vi "DG_Info.vi"(8 "error in (no error)":errorcluster) -> (0 "error out":errorcluster, 1 "Error code":i32, 2 "Number of Generators":i32, 3 "Generator Info":T1(array[cluster]) {"DG Product" items=["SRS_DG135"=1, "BME_DP01"=2, "BME_G02V3"=3, "BME_SG02V4"=4, "BME_G04"=5, "BME_G02V1"=6, "BME_G02V2"=7, "BME_SG02V1"=8, "BME_SG02V2"=9, "BME_SG02V3"=10, "BME_G03V1"=11, "BME_G03V2"=12, "BME_SG02V5"=13, "BME_G03V3"=14, "BME_G03V4"=15, "BME_SG02V6"=16, "BME_G03V5"=17, "BME_G05V1"=18, "BME_G05V2"=19, "BME_G05V3"=20, "BME_SG02V7"=21, "BME_SG02P1"=31, "BME_G03P1"=32, "BME_G05P1"=33, "BME_SG02P2"=34, "BME_G03P2"=35, "BME_SG02P3"=36, "BME_SG05P1"=37, "BME_G05P2"=38, "BME_SG05P2"=39, "BME_G05P3"=40, "BME_SG02P4"=41, "Unknown1"=42, "Unknown2"=43, "BME_SG08P1"=44]})   [LabVIEW 2009, in "POLARIS BME DG.lvlib"]
uses:
  POLARIS BME DG.lvlib
panel:
  # "NOTICE -- YOU MUST LEAVE THIS NOTICE IN PLACE.  PER THE TERMS OF THE LICENSE BELOW, YOU MAY SUBLICENSE THIS SOFTWARE \nIN ANY WAY THAT DOES NOT CONFLICT WITH THIS LICENSE.\n\n### BSD License (http://www.opensource.org/licenses/bsd-license.php) Begin ###\n \nCopyright (c) 2011, Applied Energetics, http://www.appliedenergetics.com,\n                               Richard Schwerdtfeger, <rschwerdtfeger@appliedenergetics.com>\n\nAll rights reserved.\n\nRedistribution and use in source and binary forms, with or without modification, are permitted provided that the \nfollowing conditions are met:\n\n    * Redistributions of source code must retain the above copyright notice, this list of conditions and the following disclaimer.\n    * Redistributions in binary form must reproduce the above copyright notice, this list of conditions and the following disclaimer \n       in the documentation and/or other materials provided with the distribution.\n    * Neither the name of Richard Schwerdtfeger, Applied Energetics, Inc., nor the names of its contributors may be used to \n       endorse or promote products derived from this software without specific prior written permission.\n\nTHIS SOFTWARE IS PROVIDED BY THE COPYRIGHT HOLDERS AND CONTRIBUTORS \"AS IS\" AND ANY EXPRESS OR IMPLIED WARRANTIES, \nINCLUDING, BUT NOT LIMITED TO, THE IMPLIED WARRANTIES OF MERCHANTABILITY AND FITNESS FOR A PARTICULAR PURPOSE ARE \nDISCLAIMED. IN NO EVENT SHALL THE COPYRIGHT OWNER OR CONTRIBUTORS BE LIABLE FOR ANY DIRECT, INDIRECT, INCIDENTAL,\n SPECIAL, EXEMPLARY, OR CONSEQUENTIAL DAMAGES (INCLUDING, BUT NOT LIMITED TO, PROCUREMENT OF SUBSTITUTE GOODS OR \nSERVICES; LOSS OF USE, DATA, OR PROFITS; OR BUSINESS INTERRUPTION) HOWEVER CAUSED AND ON ANY THEORY OF LIABILITY, \nWHETHER IN CONTRACT, STRICT LIABILITY, OR TORT (INCLUDING NEGLIGENCE OR OTHERWISE) ARISING IN ANY WAY OUT OF THE USE \nOF THIS SOFTWARE, EVEN IF ADVISED OF THE POSSIBILITY OF SUCH DAMAGE.\n\n### BSD License End ###"
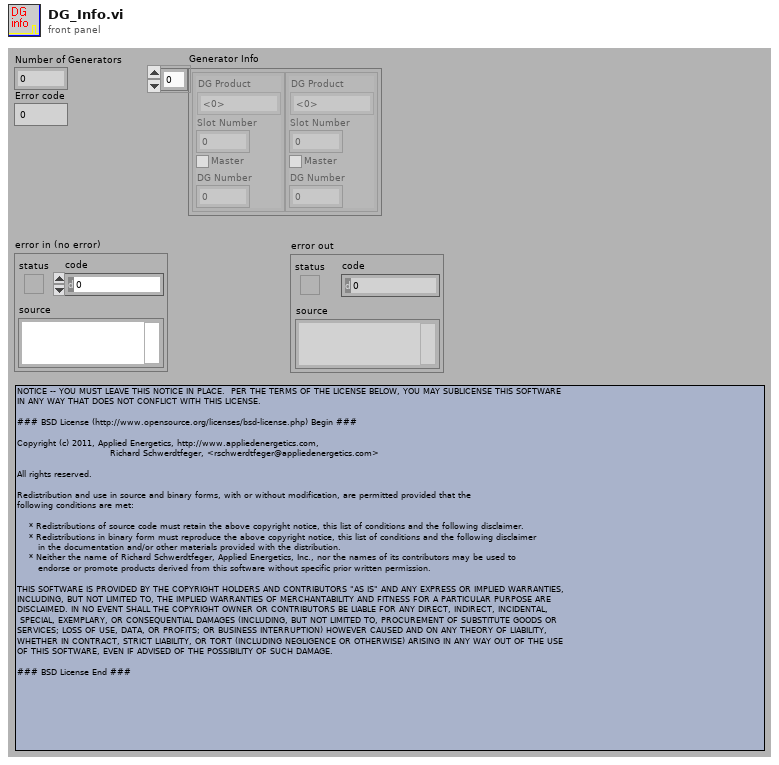
[diagram p1: front panel]
types:
  T1 = cluster{"DG Product":i32, "Slot Number":i32, "Master":bool, "DG Number":i32}[]
  T2 = cluster{"DG Product":i32, "Slot Number":i32, "Master":bool, i32}
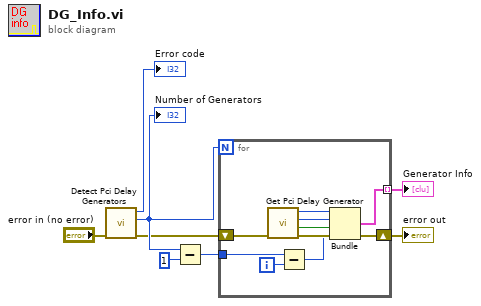
[diagram p0: block diagram]
diagram:
  n1 = call "Detect Pci Delay Generators.vi"("error in (no error)"="error in (no error)") -> ("error out"=w1:errorcluster, "Number of Generators"=w3:i32, "Error"=→"Error code":i32)  [unwired: 8 out]
  "Number of Generators" <- w3
  n2 = Subtract(x=w3, y=1) -> (x-y=w6:i32)
  n3 = for {
    N: w3 -> [_]
    tunnel: w6 -> [w16]
    tunnel: [w15] -> w8 mode=indexing
    shift-right: [w11] -> w5
    shift-left: w1 -> [w14]
    i -> [w17]
    n4 = call "Get Pci Delay Generator.vi"("error in (no error)"=w14) -> ("error out"=w11:errorcluster, "Master"=w10:bool, "Slot Number"=w12:i32, "DG Product"=w13:i32)  [unwired: 7 out]
    n5 = Subtract(x=w16, y=w17) -> (x-y=w9:i32)
    n6 = Bundle("DG Product"=w13, "Slot Number"=w12, "Master"=w10, w9) -> (w15:T2)  [unwired: 1 out]
  }
  "Generator Info" <- w8
  "error out" <- w5
